vi "10_1.vi"() -> ()   [LabVIEW 2018]
panel:
  out "Solution":dbl
  out "#3":dbl
  out "#1":dbl
  in  "Input":string
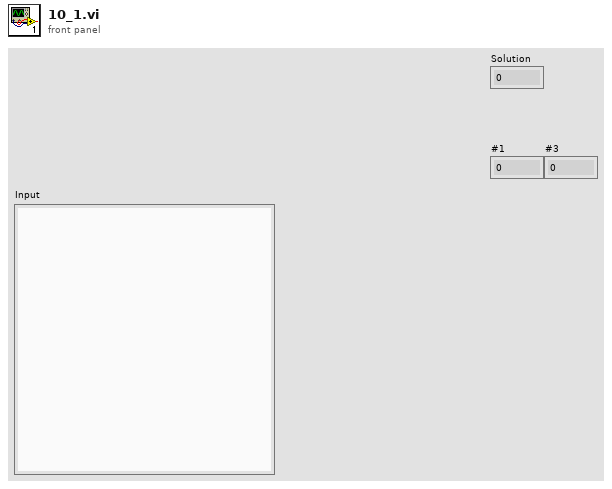
[diagram p1: front panel]
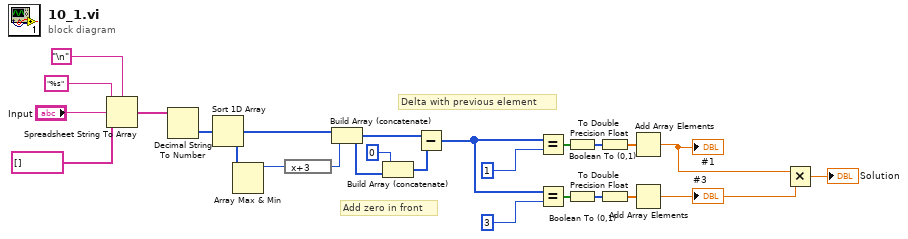
[diagram p0: block diagram]
diagram:
  # "Add zero in front"
  # "Delta with previous element"
  n1 = Spreadsheet String To Array(delimiter (Tab)="\n", format string="%s", spreadsheet string="Input", array type (2D Dbl)=string[] []) -> (array=w20:string[])
  n2 = Decimal String To Number(string=w20) -> (number=w19:i32[])  [unwired: 2 in, 1 out]
  n3 = Sort 1D Array(array=w19) -> (sorted array=w17:i32[])
  n4 = Array Max & Min(array=w17) -> (max value=w18:i32)  [unwired: 3 out]
  n5 = expression code="x+3"(w18) -> (w16:i32)
  n6 = Build Array (concatenate)(w17, w16) -> (w15:i32[])
  n7 = Build Array (concatenate)(0, w15) -> (w14:i32[])
  n8 = Subtract(x=w15, y=w14) -> (x-y=w5:i32[])
  n9 = Equal?(x=w5, y=1) -> (x = y?=w10:bool[])
  n10 = Equal?(x=w5, y=3) -> (x = y?=w6:bool[])
  n11 = Boolean To (0,1)(Boolean=w10) -> (0, 1=w9:i16[])
  n12 = Boolean To (0,1)(Boolean=w6) -> (0, 1=w7:i16[])
  n13 = To Double Precision Float(number=w9) -> (double precision float=w2:dbl[])
  n14 = To Double Precision Float(number=w7) -> (double precision float=w1:dbl[])
  n15 = Add Array Elements(numeric array=w2) -> (sum=w8:dbl)
  "#1" <- w8
  n16 = Add Array Elements(numeric array=w1) -> (sum=w3:dbl)
  "#3" <- w3
  n17 = Multiply(x=w8, y=w3) -> (x*y=→"Solution":dbl)
